vi "DAQmx.Clip AO Waveforms.vi"(8 "error in (no error)":errorcluster, 10 "AO []":waveform(dbl)[](array[waveform]), 11 "task":refnum<k21>) -> (0 "error out":errorcluster, 2 "Clipped AO []":waveform(dbl)[](array[waveform]), 3 "task out":refnum<k21>)   [LabVIEW 2019, in "DAQmx.lvclass"]
uses:
  DAQmx.lvclass
  <resource>/objmgr/daqmx.rc
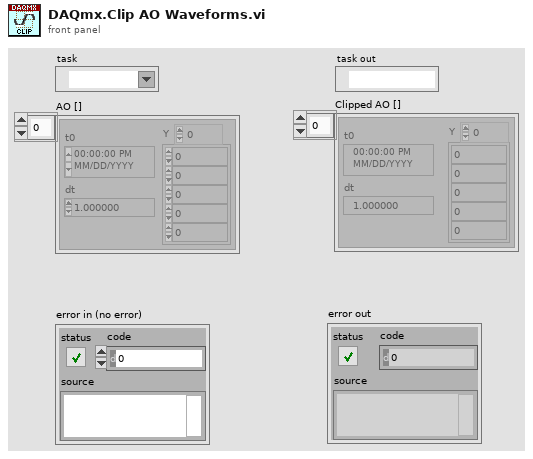
[diagram p1: front panel]
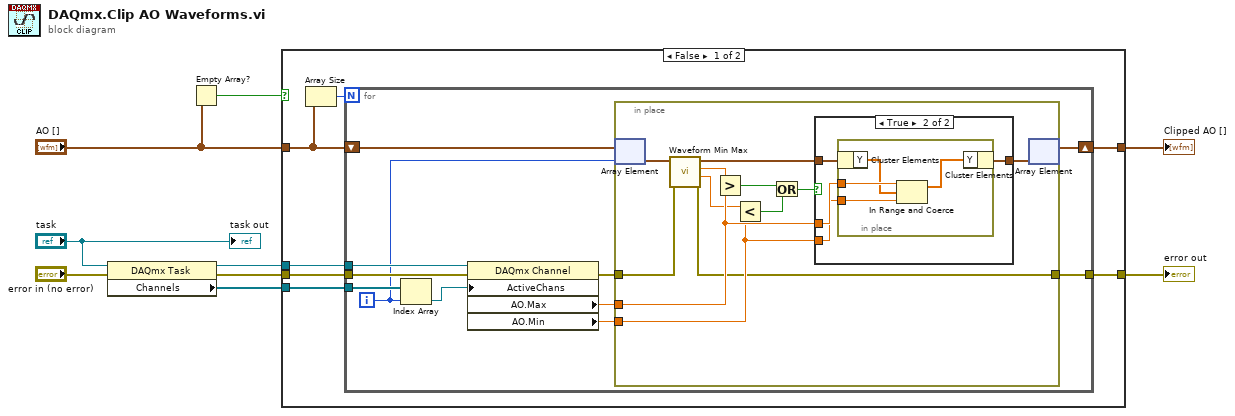
[diagram p0: block diagram]
diagram:
  n1 = property class="DAQmx Task"(reference="task", error in="error in (no error)") -> (reference out=w2:refnum<k21>, error out=w5:errorcluster, "Channels"=w6:refnum<k21>[])
  n2 = Empty Array?(array="AO []") -> (empty?=w8:bool)
  n3 = case shown="False" w8 {
    tunnel: [w16 w50] -> w9
    tunnel: "AO []" -> [w13 w50]
    tunnel: w6 -> [w14 _]
    tunnel: w5 -> [w12 w49]
    tunnel: [w11 w49] -> w3
    tunnel: w2 -> [w10 _]
    frame False {
      n4 = Array Size(array=w13) -> (size(s)=w15:i32)
      n5 = for {
        N: w15 -> [_]
        shift-right: [w26] -> w16
        shift-left: w13 -> [w27]
        tunnel: w14 -> [w24]
        tunnel: w12 -> [w22]
        tunnel: [w21] -> w11
        tunnel: w10 -> [w20]
        i -> [w19]
        n6 = Index Array(array=w24, index=w19) -> (element=w17:refnum<k21>)
        n7 = property class="DAQmx Channel"(reference=w20, error in=w22, "ActiveChans"=w17) -> (error out=w23:errorcluster, "AO.Max"=w18:dbl, "AO.Min"=w25:dbl)  [unwired: 1 out]
        n8 = in-place {
          in-place-border: w18 -> [w35]
          in-place-border: w25 -> [w30]
          in-place-border: w23 -> [w29]
          in-place-border: [w28] -> w21
          n9 = in-place-array #1(w27, w19) -> (w38:waveform(dbl))
          n10 = call <vilib>:"Waveform Min Max.vi"("error in (no error)"=w29, "waveform in"=w38) -> ("error out"=w28:errorcluster, "Y min"=w34:dbl, "Y max"=w36:dbl, "waveform out"=w37:waveform(dbl))  [unwired: 4 in, 2 out]
          n11 = Greater?(x=w36, y=w35) -> (0:w33:bool)
          n12 = Less?(x=w34, y=w30) -> (x < y?=w32:bool)
          n13 = Or(x=w33, y=w32) -> (x .or. y?=w31:bool)
          n14 = case shown="True" w31 {
            tunnel: w35 -> [_ w44]
            tunnel: w30 -> [_ w43]
            tunnel: [w40 w42] -> w39
            tunnel: w37 -> [w40 w41]
            frame False {
            }
            frame True {
              n15 = in-place {
                in-place-border: w44 -> [w48]
                in-place-border: w43 -> [w47]
                n16 = in-place-cluster #2(w41) -> ("Y"=w46:dbl[])
                n17 = In Range and Coerce(upper limit=w48, x=w46, lower limit=w47) -> (coerced(x)=w45:dbl[])  [unwired: 1 out]
                n18 = in-place-cluster #2("Y"=w45) -> (w42:waveform(dbl))
              }
            }
          }
          n19 = in-place-array #1(w39) -> (w26:waveform(dbl)[])  [unwired: 1 out]
        }
      }
    }
    frame True {
    }
  }
  "Clipped AO []" <- w9
  "error out" <- w3
  "task out" <- "task"
